vi "Generate_WayPoints_STOP_CLEAN_CV.vi"(11 "Input Cluster":T2={"Scan Rate (um/s)"=15.0, "X Start"=15.0, "X End"=15.0, "Y Start"=15.0, "Y End"=15.0, "Number of Lines"=15, "V"=15.0, "Z End"=15.0, "Approach Rate (um/s)"=15.0, "V3"=15.0, "StopMeasureDist (um)"=15.0, "CV rate (V/s)"=15.0, "V2"=15.0, "Update Position Loop Wait Time (us)"=50000, "V4"=15.0, "V1"=15.0, "Clean Time /  us"=50000, "Post Clean Pre CV time / us"=50000, "Post CV time  / us"=50000}) -> (0 "output cluster":T1)   [LabVIEW 2023]
uses:
  TypeDefs/WayPointCluster.ctl
panel:
  in  "WayPointCluster":T1
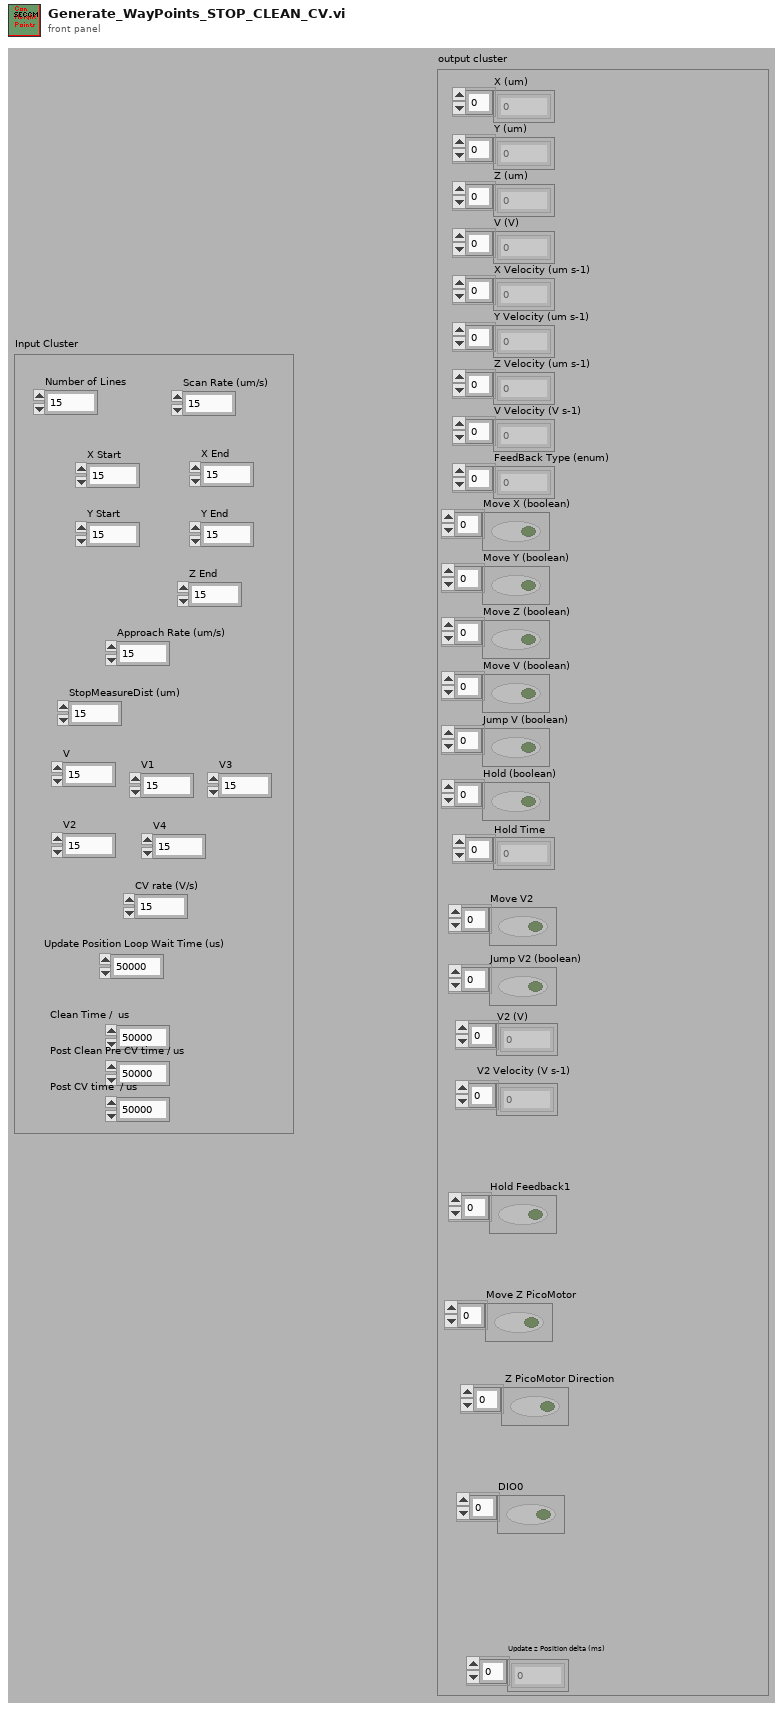
[diagram p1: front panel]
types:
  T1 = typedef "WayPointCluster.ctl" = cluster{"X (um)":dbl[], "Y (um)":dbl[], "Z (um)":dbl[], "V (V)":dbl[], "X Velocity (um s-1)":dbl[], "Y Velocity (um s-1)":dbl[], "Z Velocity (um s-1)":dbl[], "V Velocity (V s-1)":dbl[], "FeedBack Type (enum)":u16[], "Move X (boolean)":bool[], "Move Y (boolean)":bool[], "Move Z (boolean)":bool[], "Move V (boolean)":bool[], "Jump V (boolean)":bool[], "Hold (boolean)":bool[], "Hold Time":u32[], "V2 (V)":dbl[], "Move V2":bool[], "V2 Velocity (V s-1)":dbl[], "Jump V2 (boolean)":bool[], "Update z Position delta (ms)":i16[], "Hold Feedback1":bool[], "Move Z PicoMotor":bool[], " Z PicoMotor Direction":bool[], "DIO0":bool[]}
  T2 = cluster{"Scan Rate (um/s)":dbl, "X Start":dbl, "X End":dbl, "Y Start":dbl, "Y End":dbl, "Number of Lines":u32, "V":dbl, "Z End":dbl, "Approach Rate (um/s)":dbl, "V3":dbl, "StopMeasureDist (um)":dbl, "CV rate (V/s)":dbl, "V2":dbl, "Update Position Loop Wait Time (us)":u32, "V4":dbl, "V1":dbl, "Clean Time /  us":u32, "Post Clean Pre CV time / us":u32, "Post CV time  / us":u32}
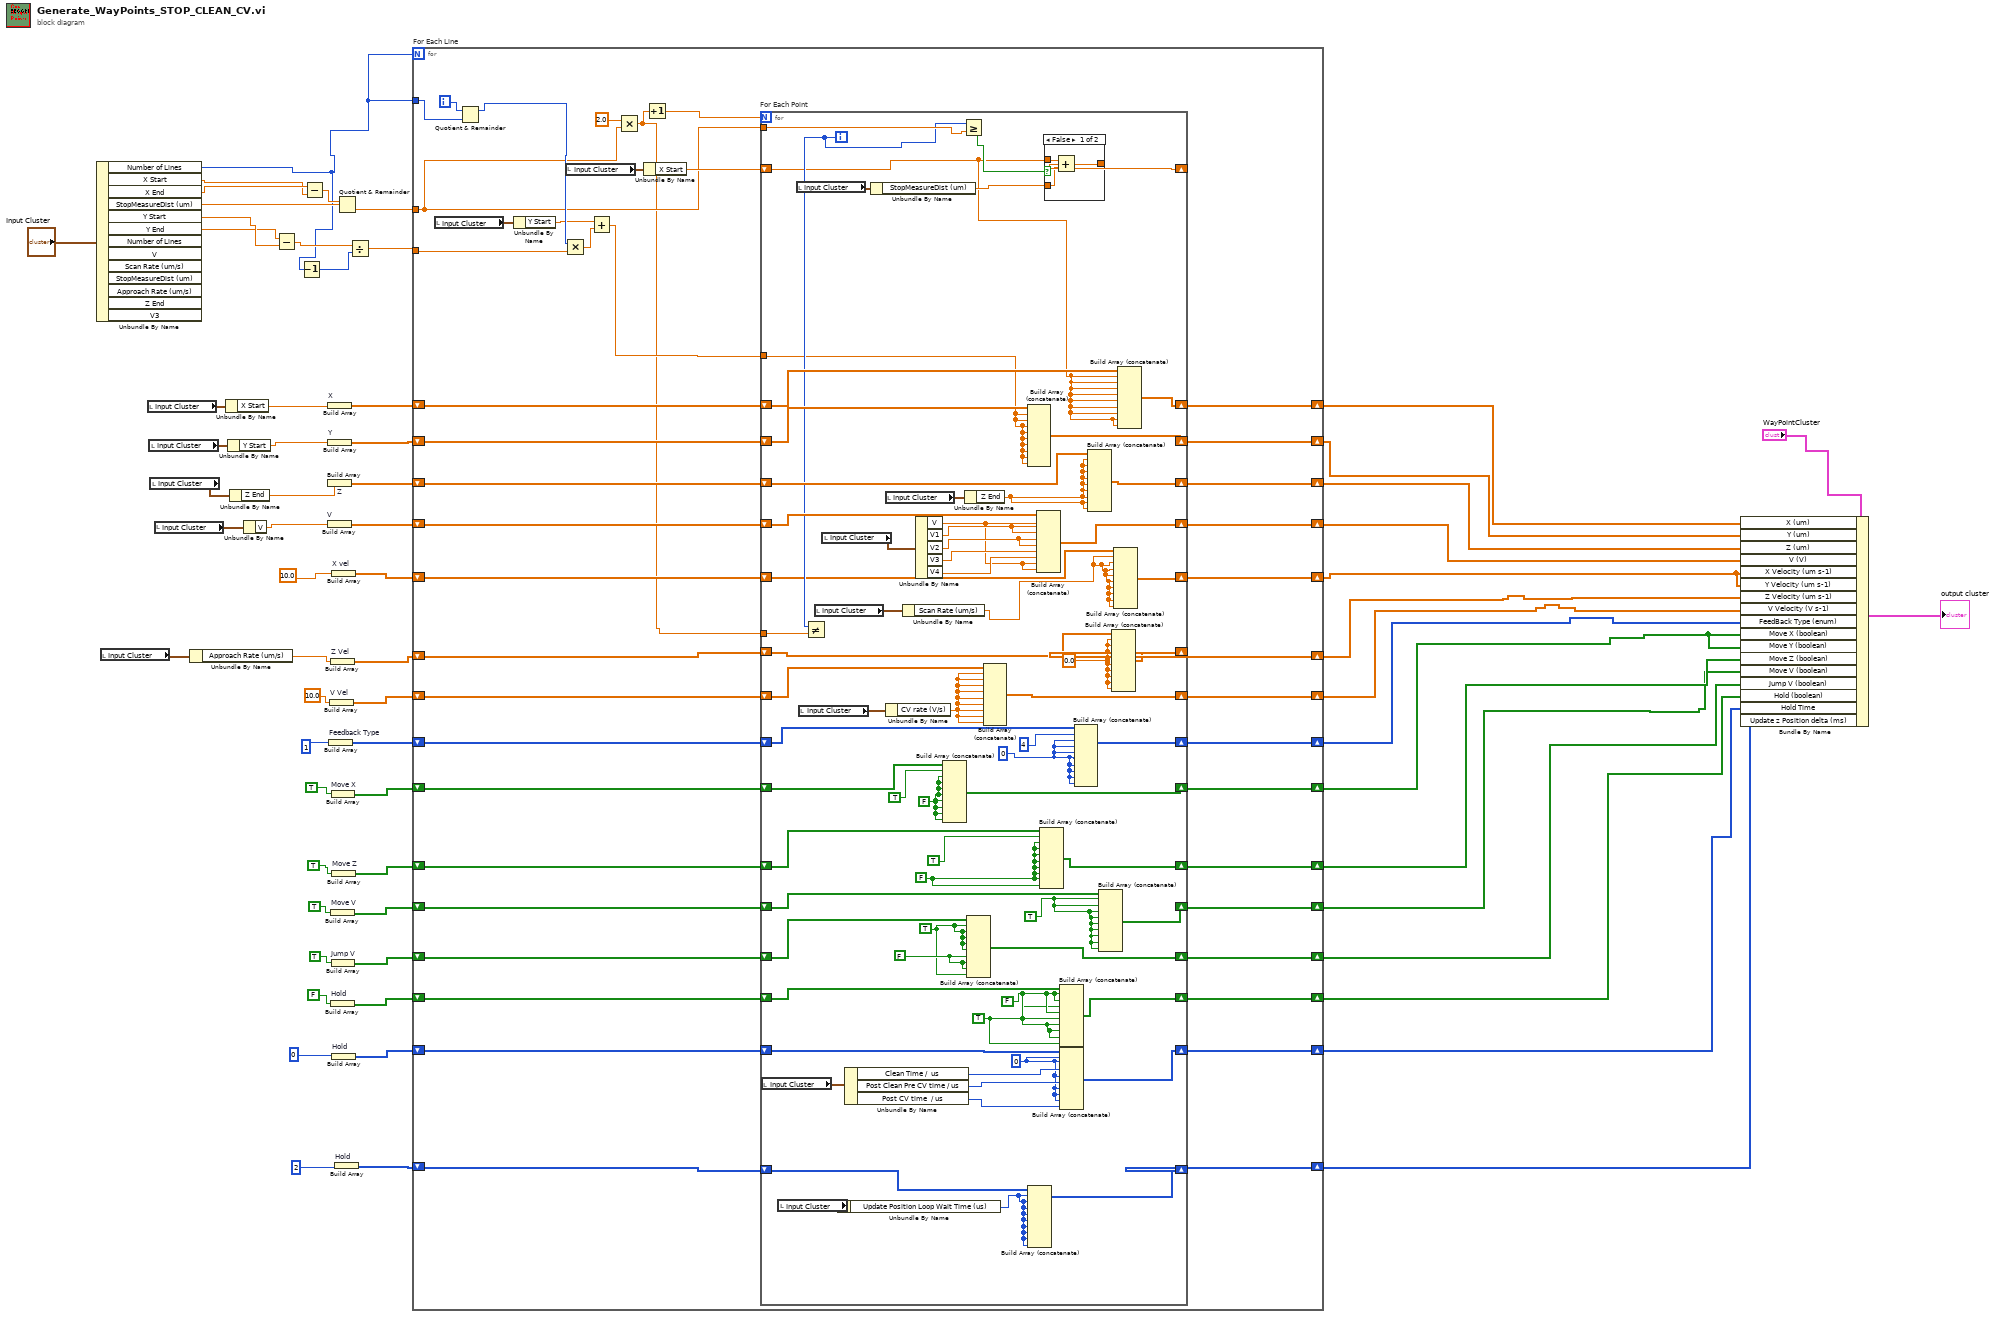
[diagram p0: block diagram]
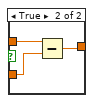
[diagram p2: hidden frame]
diagram:
  n1 = Unbundle By Name("Input Cluster") -> ("Number of Lines"=w55:u32, "X Start"=w53:dbl, "X End"=w63:dbl, "StopMeasureDist (um)"=w61:dbl, "Y Start"=w59:dbl, "Y End"=w58:dbl)  [unwired: 7 out]
  n2 = local read "Input Cluster"() -> (w34:T2)
  n3 = local read "Input Cluster"() -> (w38:T2)
  n4 = local read "Input Cluster"() -> (w37:T2)
  n5 = local read "Input Cluster"() -> (w36:T2)
  n6 = local read "Input Cluster"() -> (w35:T2)
  n7 = Unbundle By Name(w34) -> ("Approach Rate (um/s)"=w16:dbl)
  n8 = Unbundle By Name(w38) -> ("X Start"=w20:dbl)
  n9 = Unbundle By Name(w37) -> ("Y Start"=w19:dbl)
  n10 = Unbundle By Name(w36) -> ("Z End"=w9:dbl)
  n11 = Unbundle By Name(w35) -> ("V"=w18:dbl)
  n12 = Subtract(x=w58, y=w59) -> (x-y=w57:dbl)
  n13 = Decrement(x=w55) -> (x-1=w54:u32)
  n14 = Subtract(x=w63, y=w53) -> (x-y=w62:dbl)
  n15 = Build Array "V"(w18) -> (w48:dbl[])
  n16 = Build Array "X"(w20) -> (w51:dbl[])
  n17 = Build Array "Y"(w19) -> (w50:dbl[])
  n18 = Build Array "Z"(w9) -> (w49:dbl[])
  n19 = Build Array "Feedback Type"(u16 1 ("element")) -> (w44:u16[])
  n20 = Build Array "V Vel"(10.0 ("element")) -> (w45:dbl[])
  n21 = Build Array "Z Vel"(w16) -> (w46:dbl[])
  n22 = Build Array "Move V"(TRUE) -> (w41:bool[])
  n23 = Build Array "Hold"(FALSE) -> (w39:bool[])
  n24 = Build Array "Move X"(TRUE) -> (w43:bool[])
  n25 = Build Array "Jump V"(TRUE) -> (w40:bool[])
  n26 = Build Array "X vel"(10.0 ("element")) -> (w47:dbl[])
  n27 = Build Array "Move Z"(TRUE) -> (w42:bool[])
  n28 = Build Array "Hold"(u32 0 ("element")) -> (w29:u32[])
  n29 = Build Array "Hold"(u32 2 ("element")) -> (w5:u32[])
  n30 = Quotient & Remainder(x=w62, y=w61) -> (floor(x/y)=w60:dbl)  [unwired: 1 out]
  n31 = Divide(x=w57, y=w54) -> (x/y=w56:dbl)
  n32 = for "For Each Line" {
    N: w55 -> [_]
    tunnel: w60 -> [w70]
    tunnel: w55 -> [w107]
    tunnel: w56 -> [w106]
    shift-right: [w99] -> w33
    shift-left: w51 -> [w100]
    shift-right: [w86] -> w32
    shift-left: w50 -> [w98]
    shift-right: [w85] -> w31
    shift-left: w49 -> [w97]
    shift-right: [w84] -> w30
    shift-left: w48 -> [w96]
    shift-right: [w83] -> w1
    shift-left: w47 -> [w95]
    shift-right: [w82] -> w28
    shift-left: w46 -> [w94]
    shift-right: [w81] -> w27
    shift-left: w45 -> [w93]
    shift-right: [w80] -> w26
    shift-left: w44 -> [w92]
    shift-right: [w79] -> w2
    shift-left: w43 -> [w91]
    shift-right: [w78] -> w25
    shift-left: w42 -> [w90]
    shift-right: [w77] -> w24
    shift-left: w41 -> [w89]
    shift-right: [w76] -> w23
    shift-left: w40 -> [w88]
    shift-right: [w75] -> w22
    shift-left: w39 -> [w87]
    shift-right: [w67] -> w21
    shift-left: w29 -> [w68]
    shift-right: [w65] -> w4
    shift-left: w5 -> [w66]
    i -> [w108]
    n33 = local read "Input Cluster"() -> (w103:T2)
    n34 = Quotient & Remainder(x=w108, y=w107) -> (x-y*floor(x/y)=w105:u32)  [unwired: 1 out]
    n35 = Unbundle By Name(w103) -> ("Y Start"=w102:dbl)
    n36 = Multiply(x=w105, y=w106) -> (x*y=w104:dbl)
    n37 = local read "Input Cluster"() -> (w73:T2)
    n38 = Add(x=w102, y=w104) -> (x+y=w101:dbl)
    n39 = Multiply(x=2.0, y=w70) -> (x*y=w69:dbl)
    n40 = Unbundle By Name(w73) -> ("X Start"=w72:dbl)
    n41 = Increment(x=w69) -> (x+1=w71:dbl)
    n42 = for "For Each Point" {
      N: w71 -> [_]
      tunnel: w101 -> [w140]
      shift-right: [w176] -> w99
      shift-left: w100 -> [w177]
      shift-right: [w174] -> w86
      shift-left: w98 -> [w175]
      shift-right: [w172] -> w85
      shift-left: w97 -> [w173]
      shift-right: [w170] -> w84
      shift-left: w96 -> [w171]
      shift-right: [w137] -> w83
      shift-left: w95 -> [w138]
      shift-right: [w134] -> w82
      shift-left: w94 -> [w135]
      shift-right: [w131] -> w81
      shift-left: w93 -> [w132]
      shift-right: [w169] -> w80
      shift-left: w92 -> [w163]
      shift-right: [w168] -> w79
      shift-left: w91 -> [w162]
      shift-right: [w167] -> w78
      shift-left: w90 -> [w161]
      shift-right: [w166] -> w77
      shift-left: w89 -> [w160]
      shift-right: [w165] -> w76
      shift-left: w88 -> [w159]
      shift-right: [w164] -> w75
      shift-left: w87 -> [w158]
      tunnel: w69 -> [w155]
      shift-right: [w153] -> _
      shift-left: w72 -> [w141]
      tunnel: w70 -> [w152]
      shift-right: [w148] -> w67
      shift-left: w68 -> [w149]
      shift-right: [w146] -> w65
      shift-left: w66 -> [w147]
      i -> [w150]
      w121 = TRUE
      w123 = TRUE
      w128 = FALSE
      w126 = FALSE
      w110 = u16 0 ("element")
      w130 = u16 0 ("element")
      w133 = 0.0 ("element")
      w122 = FALSE
      w124 = FALSE
      w125 = TRUE
      n43 = local read "Input Cluster"() -> (w113:T2)
      n44 = local read "Input Cluster"() -> (w120:T2)
      n45 = local read "Input Cluster"() -> (w178:T2)
      n46 = local read "Input Cluster"() -> (w142:T2)
      n47 = Not Equal?(x=w150, y=w155) -> ()  [unwired: 1 out]
      n48 = local read "Input Cluster"() -> (w145:T2)
      n49 = local read "Input Cluster"() -> (w156:T2)
      n50 = Unbundle By Name(w120) -> ("Update Position Loop Wait Time (us)"=w119:u32)
      n51 = Unbundle By Name(w113) -> ("Clean Time /  us"=w112:u32, "Post Clean Pre CV time / us"=w111:u32, "Post CV time  / us"=w109:u32)
      n52 = Unbundle By Name(w178) -> ("StopMeasureDist (um)"=w154:dbl)
      n53 = local read "Input Cluster"() -> (w157:T2)
      n54 = Unbundle By Name(w142) -> ("CV rate (V/s)"=w129:dbl)
      n55 = Unbundle By Name(w145) -> ("Scan Rate (um/s)"=w136:dbl)
      n56 = Unbundle By Name(w156) -> ("V"=w114:dbl, "V1"=w118:dbl, "V2"=w117:dbl, "V3"=w116:dbl, "V4"=w115:dbl)
      n57 = Build Array (concatenate) ("X")(w162, TRUE, w128, w128, w128, w128, w128, w128, w128, w128) -> (w168:bool[])
      n58 = Greater Or Equal?(x=w150, y=w152) -> (x >= y?=w151:bool)
      n59 = Unbundle By Name(w157) -> ("Z End"=w139:dbl)
      n60 = Build Array (concatenate) ("X")(w159, w123, w123, w123, w123, w123, w124, w124, w124, w123) -> (w165:bool[])
      n61 = Build Array (concatenate) ("X")(w132, w129, w129, w129, w129, w129, w129, w129, w129, w129) -> (w131:dbl[])
      n62 = Build Array (concatenate) ("X")(w175, w140, w140, w140, w140, w140, w140, w140, w140, w140) -> (w174:dbl[])
      n63 = Build Array (concatenate) ("X")(w147, w119, w119, w119, w119, w119, w119, w119, w119, w119) -> (w146:u32[])
      n64 = Build Array (concatenate) ("X")(w171, w114, w118, w118, w117, w117, w116, w115, w114, w114) -> (w170:dbl[])
      n65 = Build Array (concatenate) ("X")(w161, TRUE, w126, w126, w126, w126, w126, w126, w126, w126) -> (w167:bool[])
      n66 = case shown="False" w151 {
        tunnel: w154 -> [w181 w184]
        tunnel: w141 -> [w180 w182]
        tunnel: [w179 w183] -> w153
        frame False {
          n67 = Add(x=w180, y=w181) -> (x+y=w179:dbl)
        }
        frame True {
          n68 = Subtract(x=w182, y=w184) -> (x-y=w183:dbl)
        }
      }
      n69 = Build Array (concatenate) ("X")(w158, w122, w122, w121, w122, w121, w122, w122, w122, w121) -> (w164:bool[])
      n70 = Build Array (concatenate) ("X")(w149, w110, w110, w112, w110, w111, w110, w110, w110, w109) -> (w148:u32[])
      n71 = Build Array (concatenate) ("X")(w163, u16 4 ("element"), w130, w130, w130, w130, w130, w130, w130, w130) -> (w169:u16[])
      n72 = Build Array (concatenate) ("X")(w173, w139, w139, w139, w139, w139, w139, w139, w139, w139) -> (w172:dbl[])
      n73 = Build Array (concatenate) ("X")(w160, w125, w125, w125, w125, w125, w125, w125, w125, w125) -> (w166:bool[])
      n74 = Build Array (concatenate) ("X")(w135, w133, w133, w133, w133, w133, w133, w133, w133, w133) -> (w134:dbl[])
      n75 = Build Array (concatenate) ("X")(w138, w136, w136, w136, w136, w136, w136, w136, w136, w136) -> (w137:dbl[])
      n76 = Build Array (concatenate) ("X")(w177, w141, w141, w141, w141, w141, w141, w141, w141, w141) -> (w176:dbl[])
    }
  }
  n77 = Bundle By Name(cluster="WayPointCluster", "X (um)"=w33, "Y (um)"=w32, "Z (um)"=w31, "V (V)"=w30, "X Velocity (um s-1)"=w1, "Y Velocity (um s-1)"=w1, "Z Velocity (um s-1)"=w28, "V Velocity (V s-1)"=w27, "FeedBack Type (enum)"=w26, "Move X (boolean)"=w2, "Move Y (boolean)"=w2, "Move Z (boolean)"=w25, "Move V (boolean)"=w24, "Jump V (boolean)"=w23, "Hold (boolean)"=w22, "Hold Time"=w21, "Update z Position delta (ms)"=w4) -> (→"output cluster":T1)
